vi "SavePedestalCalibV1729A.vi"(7 "Address":u32, 8 "error in (no error)":errorcluster, 9 "Group Name":string="Calibration", 10 "Data In":dbl[][](array[numeric]), 11 "File Handle":T1 format="%.0x") -> (0 "error out":errorcluster)   [LabVIEW 2014]
uses:
  <vilib>/addons/h5labview2/base/hid_t.ctl
  <vilib>/addons/h5labview2/base/lib_path.vi
  <vilib>/addons/h5labview2/base/H5Equery.vi
  <vilib>/addons/h5labview2/dataset/H5Dwrite.llb/H5Dwrite.xnode
  <vilib>/addons/h5labview2/group/H5G.lvlib
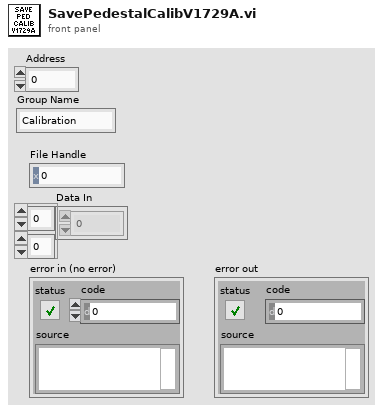
[diagram p1: front panel]
types:
  T1 = typedef "hid_t.ctl" = i32
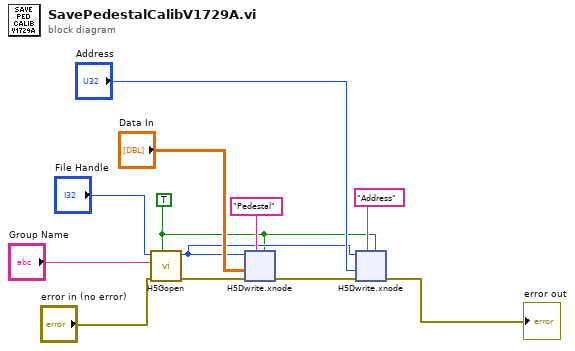
[diagram p0: block diagram]
diagram:
  w1 = TRUE ("create? (F)")
  n1 = call <vilib>:"H5Gopen.vi"("create? (F)"=w1, "error in (no error)"="error in (no error)", "name"="Group Name", "ref in"="File Handle") -> ("error out"=w9:errorcluster, "group out"=w3:T1)  [unwired: 6 in]
  n2 = xnode "H5Dwrite.xnode"("replace? (F)"=w1, "dataset name"="Pedestal", "error in (no error)"=w9, "data"="Data In", "ref in"=w3) -> ("error out"=w6:errorcluster)  [unwired: 2 in, 2 out]
  n3 = xnode "H5Dwrite.xnode"("replace? (F)"=w1, "dataset name"="Address", "error in (no error)"=w6, "data"="Address", "ref in"=w3) -> ("error out"=→"error out":errorcluster)  [unwired: 2 in, 2 out]
